vi "Shut Down.vi"(8 "error in":errorcluster, 11 "EXFO in":refnum<class "EXFO.lvclass">) -> (0 "error out":errorcluster)   [LabVIEW 2018, in "EXFO.lvlib" / "EXFO.lvclass"]
doc: "This is a static dispatch VI. It uses child methods to shutter the laser, unlock the panel controls, and free the resource. \n\nAuthor: Ron Dexter\nCompany: Luminar\nModified: 5/20/2018"
uses:
  EXFO.lvclass
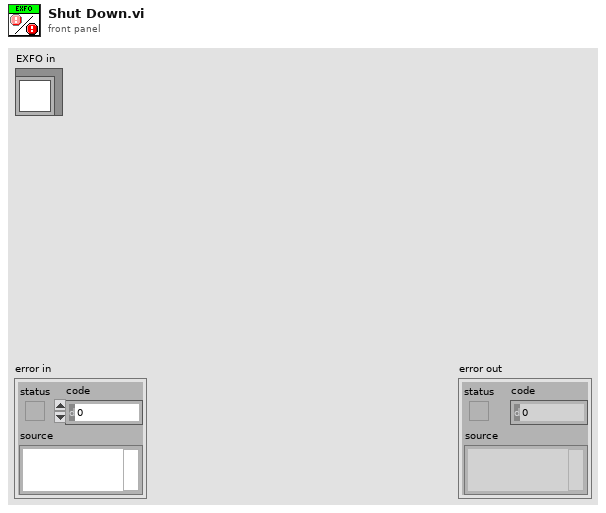
[diagram p1: front panel]
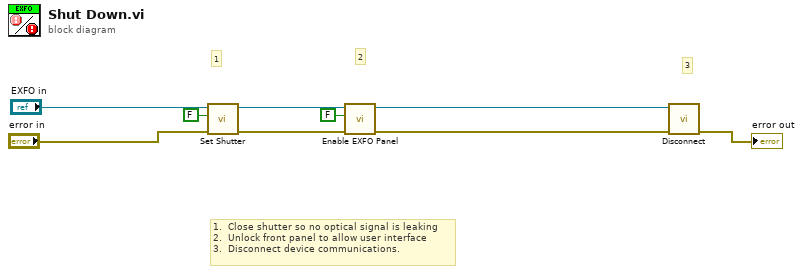
[diagram p0: block diagram]
diagram:
  # "1.  Close shutter so no optical signal is leaking\n2.  Unlock front panel to allow user interface\n3.  Disconnect device communications."
  # "3"
  # "2"
  # "1"
  n1 = call-dynamic "Set Shutter.vi"("error in (no error)"="error in", "Shutter"=FALSE, "EXFO in"="EXFO in") -> ("error out"=w3:errorcluster, "EXFO out"=w5:refnum<class "EXFO.lvclass">)  [unwired: 7 in]
  n2 = call-dynamic "Enable EXFO Panel.vi"("error in (no error)"=w3, "Lock"=FALSE, "EXFO in"=w5) -> ("error out"=w2:errorcluster, "EXFO out"=w4:refnum<class "EXFO.lvclass">)  [unwired: 7 in]
  n3 = call-dynamic "Disconnect.vi"("error in (no error)"=w2, "EXFO in"=w4) -> ("error out"=→"error out":errorcluster)  [unwired: 8 in, 1 out]
